vi "Write Motor disconnected.vi"(8 "error in (no error)":errorcluster, 10 "Motor disconnected":bool, 11 "VacuumLine in":refnum<class "VacuumLine.lvclass">) -> (0 "error out":errorcluster, 3 "VacuumLine out":refnum<class "VacuumLine.lvclass">)   [LabVIEW 2016, in "Hardware.lvlib" / "VacuumLine.lvlib" / "VacuumLine.lvclass"]
uses:
  <userlib>/Common Components/Hardware/Abstract System/VacuumLine/VacuumLine/VacuumLine.lvclass
  <userlib>/Common Components/Hardware/Abstract System/VacuumLine/VacuumLine/VacuumLine.lvclass/VacuumLine.ctl
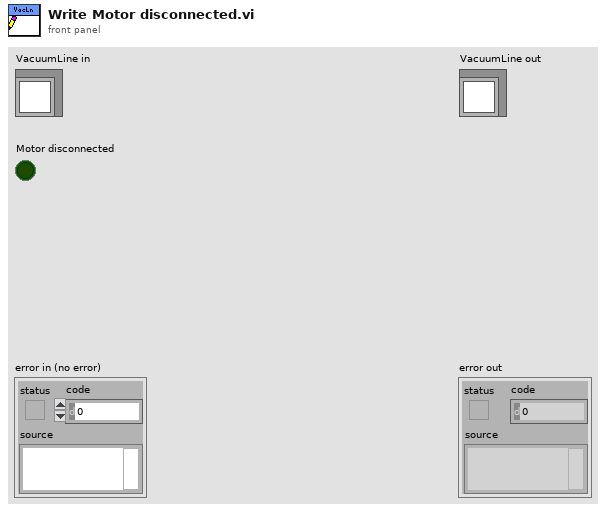
[diagram p1: front panel]
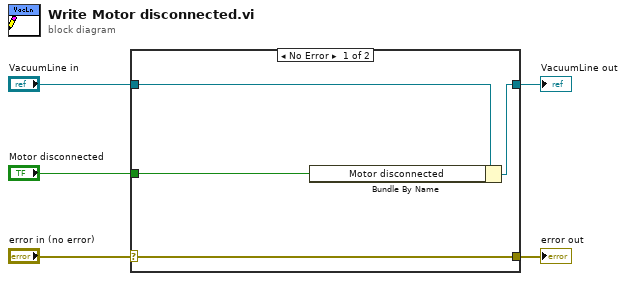
[diagram p0: block diagram]
diagram:
  n1 = case shown="No Error" "error in (no error)" {
    selector: "error in (no error)" -> [w9 w10]
    tunnel: [w9 w10] -> w4
    tunnel: [w7 w11] -> w2
    tunnel: "VacuumLine in" -> [w8 w11]
    tunnel: "Motor disconnected" -> [w6 _]
    frame No Error {
      n2 = Bundle By Name(cluster=w8, "Motor disconnected"=w6) -> (w7:refnum<class "VacuumLine.lvclass">)
    }
    frame Error {
    }
  }
  "error out" <- w4
  "VacuumLine out" <- w2
